vi "RT Loop - EPICS Control.vi"(8 "Error":errorcluster, 10 "Acquisition and Logging Configuration":T1, 11 "Message Handler":refnum<queue>) -> ()   [LabVIEW 2014]
uses:
  support/Message Queue/Message Cluster.ctl
  controls/Master Configuration.ctl
  controls/EPICS Configuration.ctl
  controls/FPGA VI Reference.ctl
  Globals/Global - Monitoring Variables.vi
  Globals/Global - All RT Loop Stop.vi
  <vilib>/Utility/error.llb/Error Cluster From Error Code.vi
  <vilib>/RVI Host/nirviSupport.llb/nirviErrorClusterFromErrorCode.vi
  <vilib>/rvi/errors/niLvFpgaAdjustHostInterfaceError.vi
  <vilib>/rvi/interface/nirviMethod/nirviMethod.xnode
  <vilib>/nisyscfg/nisyscfg.lvlib
  <vilib>/rvi/interface/nirviMethod/StockFPGA_InlinedMethodWaitForMultipleIRQ.vi
  <vilib>/FPGAPlugInAG/Dynamic/niLvFpga_WaitOnIrq_Dynamic.vi
  <vilib>/FPGAPlugInAG/Dynamic/niLvFpga_AcknowledgeIrq_Dynamic.vi
  support/Message Queue/Message Queue.lvlib
panel:
  out "Error":errorcluster
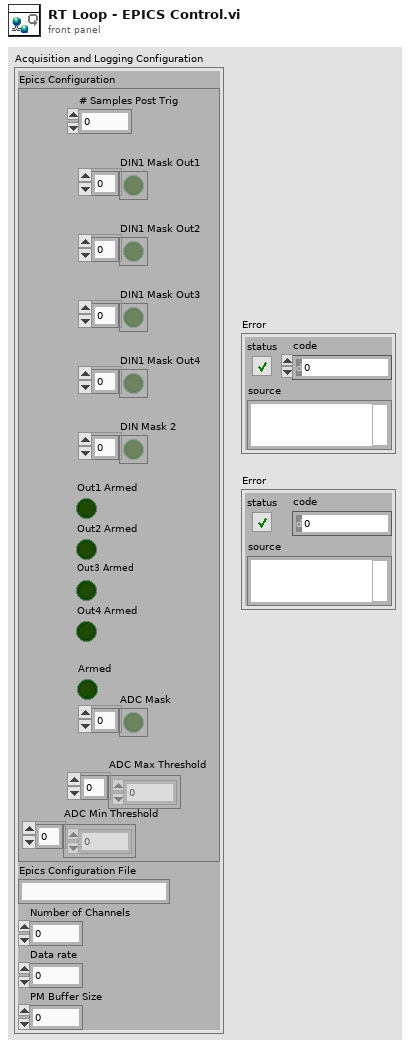
[diagram p1: front panel]
types:
  T1 = typedef "Master Configuration.ctl" = cluster{"Epics Configuration":T2, "Epics Configuration File":string, "Number of Channels":u8, "Data rate":u32, "PM Buffer Size":u32}
  T2 = typedef "EPICS Configuration.ctl" = cluster{"DIN1 Mask Out1":bool[], "# Samples Post Trig":u32, "Armed":bool, "ADC Mask":bool[], "ADC Max Threshold":dbl[], "ADC Min Threshold":dbl[], "DIN Mask 2":bool[], "DIN1 Mask Out2":bool[], "DIN1 Mask Out3":bool[], "DIN1 Mask Out4":bool[], "Out3 Armed":bool, "Out1 Armed":bool, "Out4 Armed":bool, "Out2 Armed":bool}
  T3 = typedef "FPGA VI Reference.ctl" = refnum<k20>
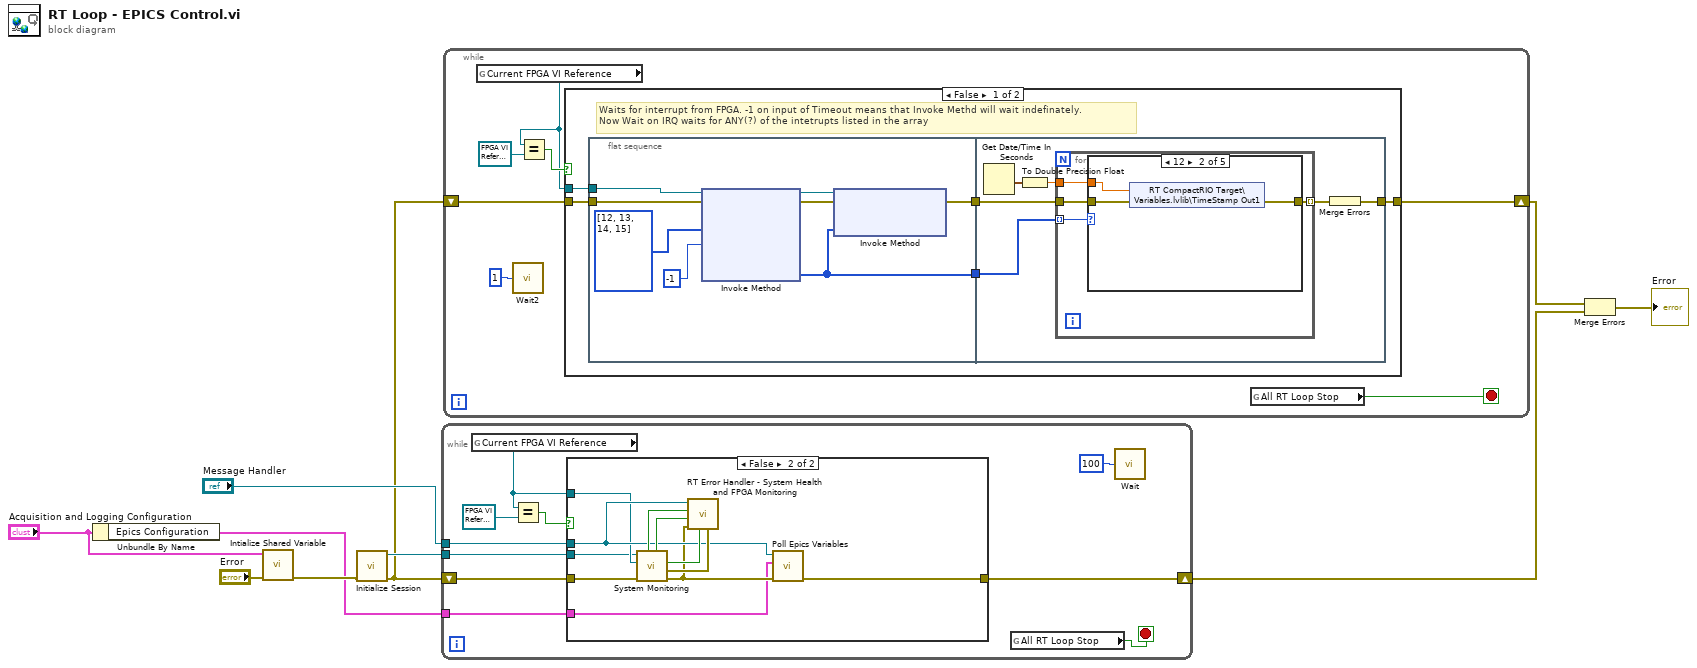
[diagram p0: block diagram]
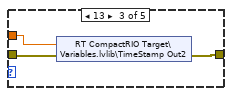
[diagram p3: hidden frame]
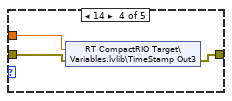
[diagram p4: hidden frame]
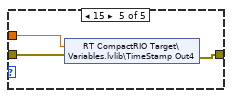
[diagram p5: hidden frame]
diagram:
  n1 = Unbundle By Name("Acquisition and Logging Configuration") -> ("Epics Configuration"=w2:T2)
  n2 = call "Intialize Shared Variable.vi"("error in (no error)"="Error", "Master Configuration"="Acquisition and Logging Configuration") -> ("error out"=w7:errorcluster)  [unwired: 9 in]
  n3 = call <vilib>:"Initialize Session.vi"("error in (no error)"=w7) -> ("error out"=w5:errorcluster, "Session out"=w6:refnum<k21>)  [unwired: 9 in]
  n4 = while {
    tunnel: "Message Handler" -> [w16]
    shift-right: [w17] -> w9
    shift-left: w5 -> [w18]
    tunnel: w6 -> [w12]
    tunnel: w2 -> [w11]
    stop <- w19 stop-if-true
    n5 = global read "Global - Monitoring Variables.vi" "Current FPGA VI Reference"() -> (w13:T3)
    n6 = Equal?(x=w13, y=T3 refnum ("Current FPGA VI Reference")) -> (x = y?=w14:bool)
    n7 = case shown="False" w14 {
      tunnel: w18 -> [w21 w25]
      tunnel: [w21 w24] -> w17
      tunnel: w16 -> [_ w28]
      tunnel: w13 -> [_ w27]
      tunnel: w12 -> [_ w26]
      tunnel: w11 -> [_ w22]
      frame True {
      }
      frame False {
        n8 = call "System Monitoring.vi"("Error"=w25, "Current FPGA VI Reference"=w27, "Refnum in"=w26) -> ("Error"=w23:errorcluster, "FPGA Error"=w32:errorcluster, "Different Channel Count"=w31:bool, "DMA FIFO Full"=w30:bool, "Sample Gated"=w29:bool)  [unwired: 2 in, 1 out]
        n9 = call "RT Error Handler - System Health and FPGA Monitoring.vi"("FPGA Error (FPGA)"=w32, "Different Channel Count (FPGA)"=w31, "error in (no error)"=w23, "DMA FIFO Full (FPGA)"=w30, "Sample Gated (FPGA)"=w29, "Message Queue"=w28) -> ()  [unwired: 5 in, 1 out]
        n10 = call "Poll Epics Variables.vi"("error in (no error)"=w23, "Epics Initial Configuration"=w22, "Queue in"=w28) -> ("error out"=w24:errorcluster)  [unwired: 8 in]
      }
    }
    n11 = global read "Global - All RT Loop Stop.vi" "All RT Loop Stop"() -> (w19:bool)
    n12 = call "Wait"("Count(mSec)"=u32 100) -> ()  [unwired: 1 out]
  }
  n13 = while {
    shift-right: [w33] -> w3
    shift-left: w5 -> [w34]
    stop <- w39 stop-if-true
    n14 = global read "Global - Monitoring Variables.vi" "Current FPGA VI Reference"() -> (w36:T3)
    n15 = call "Wait2"("Count(mSec)"=u32 1) -> ()  [unwired: 1 out]
    n16 = Equal?(x=w36, y=T3 refnum ("Current FPGA VI Reference")) -> (x = y?=w37:bool)
    n17 = case shown="False" w37 {
      tunnel: w36 -> [w44 _]
      tunnel: w34 -> [w42 w76]
      tunnel: [w41 w76] -> w33
      frame False {
        # "Waits for interrupt from FPGA. -1 on input of Timeout means that Invoke Methd will wait indefinately.\nNow Wait on IRQ waits for ANY(?) of the intetrupts listed in the array"
        n18 = flat-sequence {
          tunnel: w44 -> [w52]
          tunnel: [w47] -> w43
          tunnel: w42 -> [w51]
          tunnel: [w45] -> w40
          tunnel: w43 -> [w56]
          tunnel: [w53] -> w41
          tunnel: w40 -> [w57]
          frame #0 {
            n19 = xnode "Invoke Method"("FPGA VI Reference In"=w52, "error in"=w51, "IRQ Number(s)"=i32[] [12, 13, 14, 15], "Timeout (ms)"=-1) -> ("FPGA VI Reference Out"=w49:T3, "error out"=w48:errorcluster, "IRQ(s) Asserted"=w45:i32[])  [unwired: 1 out]
            n20 = xnode "Invoke Method"("FPGA VI Reference In"=w49, "error in"=w48, "IRQ Number(s)"=w45) -> ("error out"=w47:errorcluster)  [unwired: 1 out]
          }
          frame #1 {
            n21 = Get Date/Time In Seconds() -> (seconds since 1Jan1904=w58:timestamp)
            n22 = To Double Precision Float(number=w58) -> (double precision float=w55:dbl)
            n23 = for {
              tunnel: w57 -> [w61] mode=indexing
              tunnel: w56 -> [w59]
              tunnel: [w62] -> w54 mode=indexing
              tunnel: w55 -> [w60]
              n24 = case shown="12" w61 {
                tunnel: [w63 w66 w69 w72 w75] -> w62
                tunnel: w60 -> [_ w65 w68 w71 w74]
                tunnel: w59 -> [w63 w64 w67 w70 w73]
                frame 0, Default {
                }
                frame 12 {
                  n25 = shared-variable "RT CompactRIO Target\\Variables.lvlib\\TimeStamp Out1"(w65, error in=w64) -> (error out=w66:errorcluster)
                }
                frame 13 {
                  n26 = shared-variable "RT CompactRIO Target\\Variables.lvlib\\TimeStamp Out2"(w68, error in=w67) -> (error out=w69:errorcluster)
                }
                frame 14 {
                  n27 = shared-variable "RT CompactRIO Target\\Variables.lvlib\\TimeStamp Out3"(w71, error in=w70) -> (error out=w72:errorcluster)
                }
                frame 15 {
                  n28 = shared-variable "RT CompactRIO Target\\Variables.lvlib\\TimeStamp Out4"(w74, error in=w73) -> (error out=w75:errorcluster)
                }
              }
            }
            n29 = Merge Errors(w54) -> (w53:errorcluster)
          }
        }
      }
      frame True {
      }
    }
    n30 = global read "Global - All RT Loop Stop.vi" "All RT Loop Stop"() -> (w39:bool)
  }
  n31 = Merge Errors(w3, w9) -> (→"Error":errorcluster)
